vi "Yale Set Gain.vi"() -> (0 "Error":bool)   [LabVIEW 2009]
doc: "This VI writes to hardware to set the desired gain on a Yale card. The device, channel, and gain information is taken from the QCA Global."
uses:
  QCA Global.vi
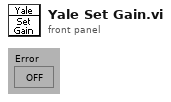
[diagram p1: front panel]
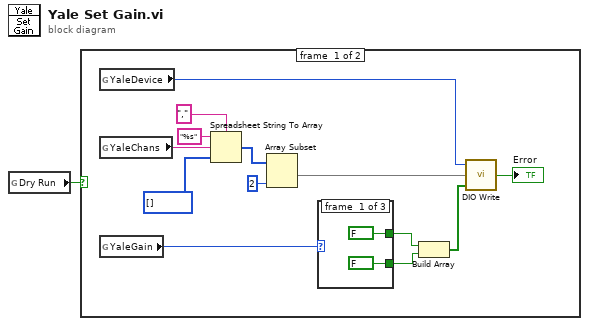
[diagram p0: block diagram]
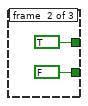
[diagram p2: hidden frame]
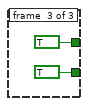
[diagram p3: hidden frame]
diagram:
  n1 = global read "QCA Global.vi" "Dry Run"() -> (w1:bool)
  n2 = case shown="False" w1 {
    frame #0 {
      n3 = global read "QCA Global.vi" "YaleDevice"() -> (w3:i16)
      n4 = global read "QCA Global.vi" "YaleChans"() -> (w14:string)
      n5 = global read "QCA Global.vi" "YaleGain"() -> (w8:i32)
      n6 = Spreadsheet String To Array(delimiter (Tab)="," ("regular expression"), format string="%s", spreadsheet string=w14, array type (2D Dbl)=i32[] [] ("Array Constant")) -> (array=w10:i32[])
      n7 = Array Subset(array=w10, length=2 ("Array Length")) -> (w4:i32[])  [unwired: 1 in]
      n8 = case shown="0, Default" w8 {
        tunnel: [FALSE TRUE TRUE] -> w5
        tunnel: [FALSE FALSE TRUE] -> w6
        frame #0 {
        }
        frame #1 {
        }
        frame #2 {
        }
      }
      n9 = Build Array(w5, w6) -> (w7:bool[])
      n10 = call "DIO Write.vi"("Data"=w7, "Channels"=w4, "device"=w3) -> ("Error"=→"Error":bool)
    }
    frame #1 {
    }
  }
